vi "ERA_Trigger.vi"(6 "Graph":bool=TRUE, 7 "Threshold":dbl, 8 "Error In":errorcluster, 11 "Data In":waveform(dbl)[](array[waveform])) -> (0 "Error Out":errorcluster, 1 "Ind_end":i32, 2 "Ind_begin":i32, 3 "Data Out":waveform(dbl)[](array[waveform]), 4 "Energy Graph":waveform(dbl)[](graph))   [LabVIEW 2017, in "AppPlugins.lvlib" / "EraPlugin.lvclass"]
uses:
  EraPlugin.lvclass
  <vilib>/Analysis/NI_AALPro.lvlib
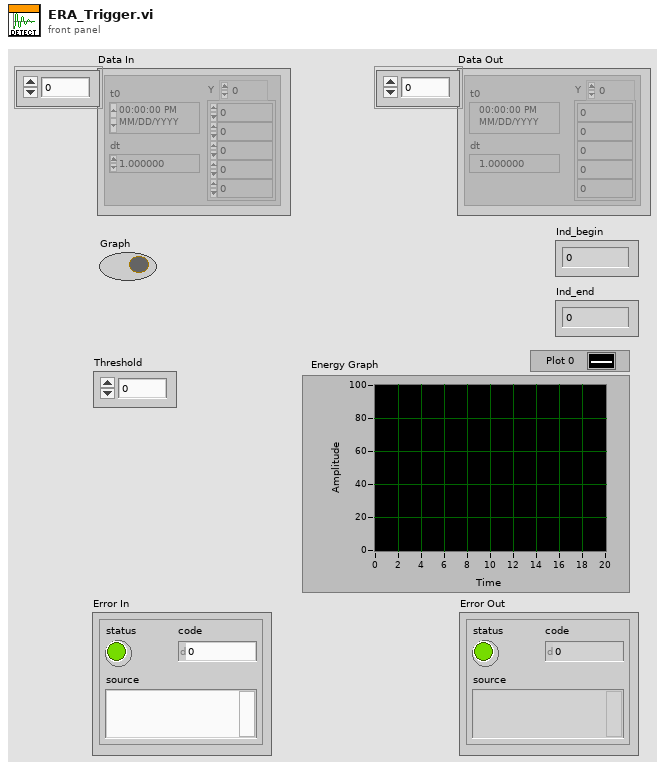
[diagram p1: front panel]
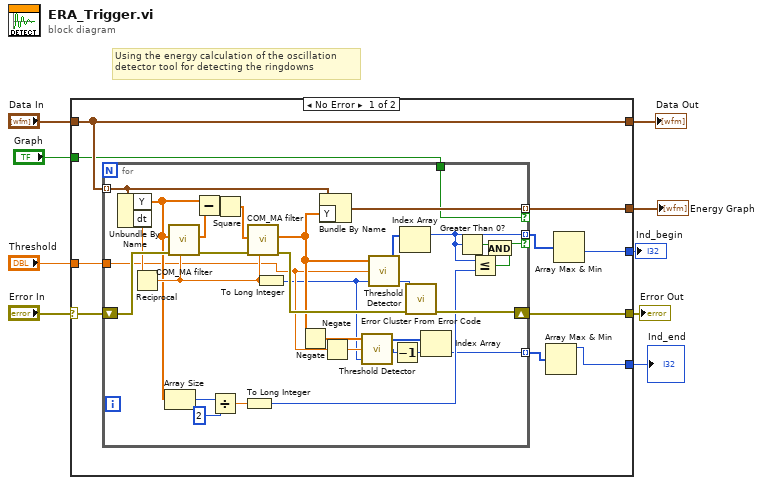
[diagram p0: block diagram]
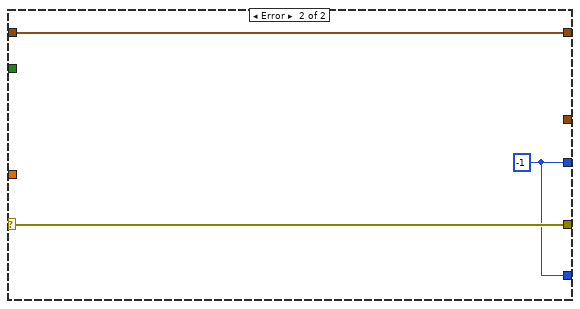
[diagram p2: hidden frame]
diagram:
  # "Using the energy calculation of the oscillation \ndetector tool for detecting the ringdowns"
  n1 = case shown="No Error" "Error In" {
    selector: "Error In" -> [w16 w53]
    tunnel: [w19 w52] -> w9
    tunnel: "Data In" -> [w17 w54]
    tunnel: "Threshold" -> [w18 _]
    tunnel: [w17 w54] -> w5
    tunnel: [w15 w53] -> w4
    tunnel: [w14 _] -> w3
    tunnel: "Graph" -> [w13 _]
    tunnel: [w10 w52] -> w1
    frame No Error {
      n2 = for {
        tunnel: w17 -> [w45] mode=indexing
        tunnel: [w44] -> w14 mode=indexing if=w38
        tunnel: w18 -> [w26]
        tunnel: [w31] -> w12 mode=indexing if=w37
        shift-right: [w40] -> w15
        shift-left: w16 -> [w51]
        tunnel: w13 -> [w38]
        tunnel: [w22] -> w11 mode=indexing
        n3 = Unbundle By Name(w45) -> ("Y"=w35:dbl[], "dt"=w49:dbl)
        n4 = Reciprocal(x=w49) -> (1/x=w43:dbl)
        n5 = Array Size(array=w35) -> (size(s)=w34:i32)
        n6 = call "COM_MA filter.vi"("Fs"=w43, "Error In"=w51, "Data In"=w35) -> ("Error Out"=w41:errorcluster, "Data Out"=w48:dbl[])  [unwired: 7 in]
        n7 = Subtract(x=w35, y=w48) -> (x-y=w47:dbl[])
        n8 = Divide(x=w34, y=2) -> (x/y=w32:dbl)
        n9 = Square(x=w47) -> (x^2=w46:dbl[])
        n10 = To Long Integer(number=w32) -> (32bit integer=w29:i32)
        n11 = call "COM_MA filter.vi"("Fs"=w43, "Error In"=w41, "Data In"=w46) -> ("Error Out"=w50:errorcluster, "Data Out"=w28:dbl[])  [unwired: 7 in]
        n12 = To Long Integer(number=w43) -> (32bit integer=w24:i32)
        n13 = Negate(x=w28) -> (-x=w27:dbl[])
        n14 = Bundle By Name(cluster=w45, "Y"=w28) -> (w44:waveform(dbl))
        n15 = Negate(x=w26) -> (-x=w25:dbl)
        n16 = call <vilib>:"Threshold Detector.vi"("width"=w24, "threshold"=w25, "X"=w27) -> ("count"=w20:i32, "Indices"=w23:i32[])  [unwired: 1 out]
        n17 = call <vilib>:"Threshold Detector.vi"("width"=w24, "threshold"=w26, "X"=w28) -> ("error"=w39:i32, "Indices"=w42:i32[])  [unwired: 1 out]
        n18 = Decrement(x=w20) -> (x-1=w21:i32)
        n19 = Index Array(array=w42) -> (element=w31:i32)  [unwired: 1 in]
        n20 = call <vilib>:"Error Cluster From Error Code.vi"("error in (no error)"=w50, "error code (0)"=w39) -> ("error out"=w40:errorcluster)  [unwired: 7 in]
        n21 = Index Array(array=w23, index=w21) -> (element=w22:i32)
        n22 = Greater Than 0?(x=w31) -> (x > 0?=w30:bool)
        n23 = Less Or Equal?(x=w31, y=w29) -> (x <= y?=w36:bool)
        n24 = And(x=w30, y=w36) -> (x .and. y?=w37:bool)
      }
      n25 = Array Max & Min(array=w11) -> (max value=w10:i32)  [unwired: 3 out]
      n26 = Array Max & Min(array=w12) -> (min value=w19:i32)  [unwired: 3 out]
    }
    frame Error {
      w52 = -1
    }
  }
  "Ind_begin" <- w9
  "Data Out" <- w5
  "Error Out" <- w4
  "Energy Graph" <- w3
  "Ind_end" <- w1
